vi "testExecution_Module.vi"(9 "Motion Cfg File path":path=path "C:/Users/Public/Documents/UCAR/APAR Board Test/SupportFiles/Motion64.ini", 10 "Cfg File path":path=path "C:/Users/Public/Documents/UCAR/APAR Board Test/SupportFiles/aparConfig.ini", 11 "MessageQues":T1) -> ()   [LabVIEW 2019]
doc: "This VI is a simple state machine that has a message que so it can be controlled by external processes.\nIt also has a control with all the messages ques in the calling application that it needs to send messages to.\n\nThe concept is to have many parallel VIs like this one. This VI should be a cohesive process. This could cut down on it's size and complexity.\n\nBolder Software LLC"
uses:
  Support/MessageQue/VXM Main Test App/MultipleMessageQues vxm.ctl
  Support/MessageQue/MessageQue.ctl
  Support/MessageQue/MessageCluster.ctl
  Classes/aparCfg/aparCfg.lvclass
  Classes/ArrayController/ArrayController.lvclass
  Classes/CopperMountain/C4209 PNA.lvclass
  Classes/Sequence/Sequence.lvclass
  Classes/Datalog/DataLog.lvclass
  Classes/SendMessage/SendMessage.lvclass
  Classes/MotionComm/MotionComm.lvclass
  UI temporary dialogs and VIs/Mode1TestProperties.ctl
  Classes/Sequence/SequenceSubvis/RF Direction.ctl
  Classes/DataLogRaster/DataLogRaster.lvclass
  C:/Users/MWUser/Desktop/GItHub/mmWave_Scanner/LVSource/Classes/Datalog/DataLog.lvclass
  VXM Public API/mmWaveAxis.ctl
  UI temporary dialogs and VIs/Mode2TestProperties.ctl
  UI temporary dialogs and VIs/Mode3TestProperties.ctl
  Support/MessageAPI/UIMessage.ctl
  Support/MessageQue/MessageQue.lvlib
  Classes/FileMerge/FileMerge.lvclass
  Classes/VXMCfg/VXMCfg.lvclass
panel:
  out "Seq Step":string
  out "i":i32
  out "Command":string
  out "error out":errorcluster
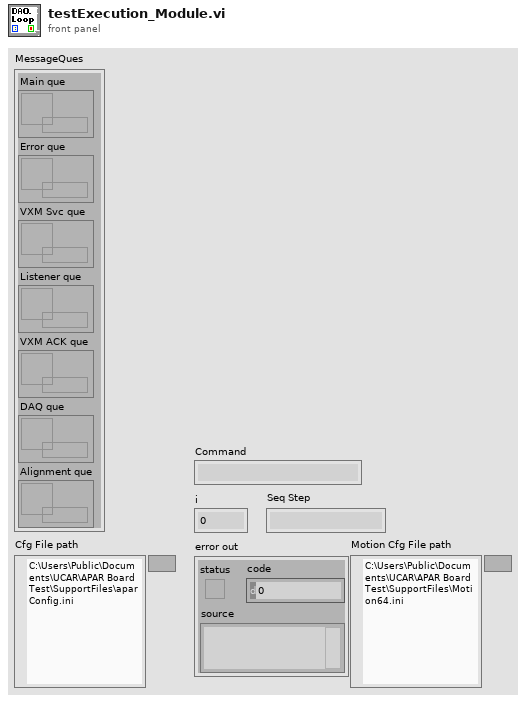
[diagram p1: front panel]
types:
  T1 = typedef "MultipleMessageQues vxm.ctl" = cluster{"Main que":T2, "Error que":T2, "VXM Svc que":T2, "Listener que":T2, "VXM ACK que":T2, "DAQ que":T2, "Alignment que":T2}
  T2 = typedef "MessageQue.lvlib/MessageQue.ctl" = refnum<queue>
  T3 = cluster{"aparCfg":refnum<class "aparCfg.lvclass">, "AC":refnum<class "ArrayController.lvclass">, "PNA":refnum<class "C4209 PNA.lvclass">, "Sequence":refnum<class "Sequence.lvclass">, "DataLog":refnum<class "DataLog.lvclass">, "UI Msg":refnum<class "SendMessage.lvclass">, "Motion ACK":refnum<class "MotionComm.lvclass">}
  T4 = typedef "UIMessage.ctl" = cluster{"EventCode":i32, "Numeric":dbl, "String":string, "Variant":variant}
  T5 = typedef "ACConfig.ctl" = cluster{"Board 1 alias":string, "Board 1 Enable":bool, "Board 2 alias":string, "Board 2 Enable":bool}
  T6 = typedef "N5222AConfig.ctl" = cluster{"ResourceName":string, "Enable":bool, "Channel":i32, "CalFileName":string, "MeasName":string, "TempDatFile":string, "Power, dBm":dbl, "NumPoints":i32, "Start Freq, Hz":dbl, "Stop Freq, Hz":dbl, "NumAverages":i32, "Sweep Type":i32, "IF Bandwidth":dbl}
  T7 = typedef "seqConfig.ctl" = cluster{"TempXMLFilePath":path, "Motion":bool}
  T8 = typedef "RunTest.ctl" = cluster{"FileNameRoot":string, "MergeFilePath":path, "Merge":bool}
  T9 = typedef "DataLogConfig.ctl" = cluster{"FilePath":path}
  T10 = typedef "sub-syst.n.ctl" = cluster{"Addr":string, "Enable":bool, "X scale eng./step":dbl, "Y scale eng./step":dbl, "Z scale eng./step":dbl, "T scale eng./step":dbl, "X units":string, "Y units":string, "Z units":string, "T units":string, "X Jog":dbl, "Y Jog":dbl, "Z Jog":dbl, "T Jog":dbl, "X-1 Name":string, "Y-2 Name":string, "Z-3 Name":string, "T-4 Name":string, "VXM (1-4)":i32}
  T11 = typedef "mmWaveAxis.ctl" = string
  T12 = typedef "Mode1TestProperties.ctl" = cluster{"Probe Horizontal Polarization":bool, "Probe Vertical Polarization":bool, "Data File Name":string, "RF In/Out of antenna":T13, "Raster XY Points":cluster{"X mm":dbl, "Y mm":dbl}[]}
  T13 = typedef "RF Direction.ctl" = enum16{"Tx - RF In", "Rx - RF Out"}
  T14 = typedef "Mode2TestProperties.ctl" = cluster{"Probe Horizontal Polarization":bool, "Probe Vertical Polarization":bool, "Upload TR Module file":path, "Data File Name":string, "RF In/Out of antenna":T13, "RT3 Positions, degrees":dbl[]}
  T15 = typedef "Mode3TestProperties.ctl" = cluster{"Probe Horizontal Polarization":bool, "Probe Vertical Polarization":bool, "Upload TR Module file":path, "Data File Name":string, "RF In/Out of antenna":T13}
  T16 = typedef "DataLog.lvclass/SearchableTag.ctl" = cluster{"Module, 0-63":i32, "RF Direction Tx0":T13, "Polarization, V0 H1":T17, "AO-64 Array":dbl[]}
  T17 = typedef "PolarizationSelect.ctl" = enum16{"Vertical", "Horizontal"}
  T18 = typedef "PatchNewTestStep.ctl" = cluster{"RF In/Out":T13, "TR Module/Raster":i32, "Polarization":T17, "Position":T19[]}
  T19 = typedef "singleAxisMoveDef.ctl" = cluster{"mmWave Axis":T11, "eng. value":dbl}
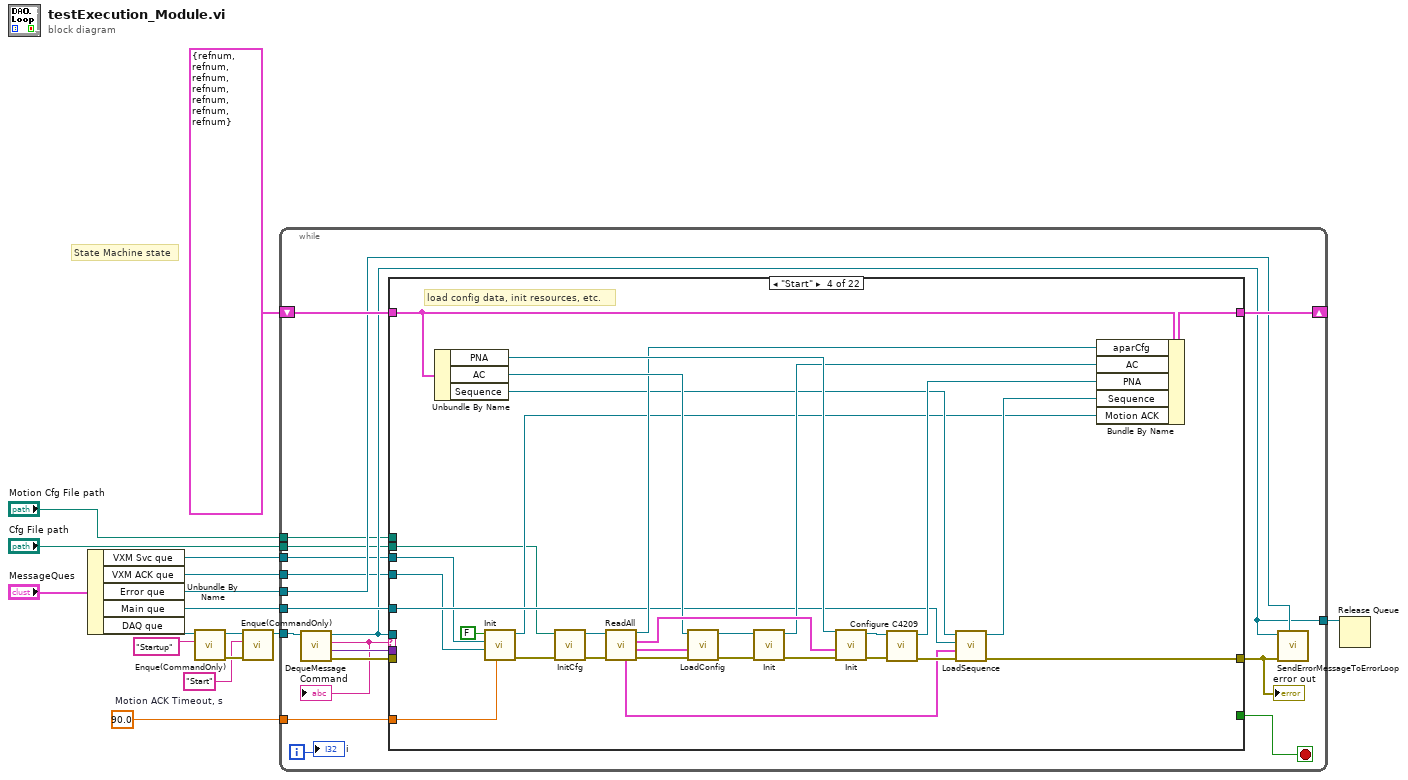
[diagram p0: block diagram]
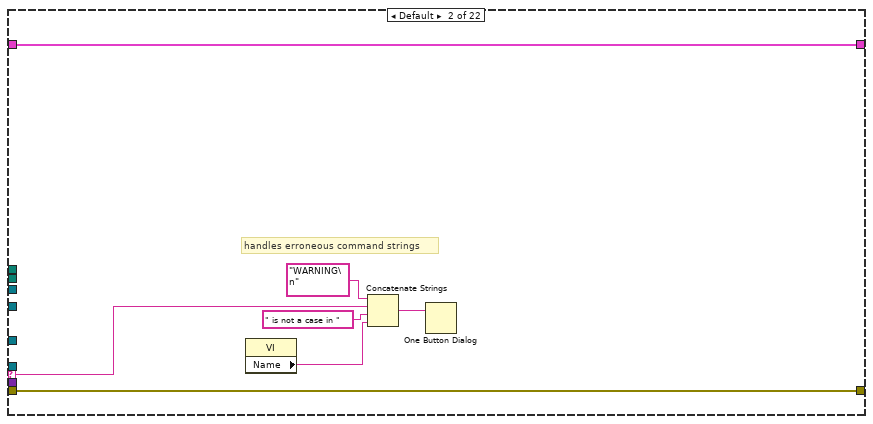
[diagram p3: hidden frame]
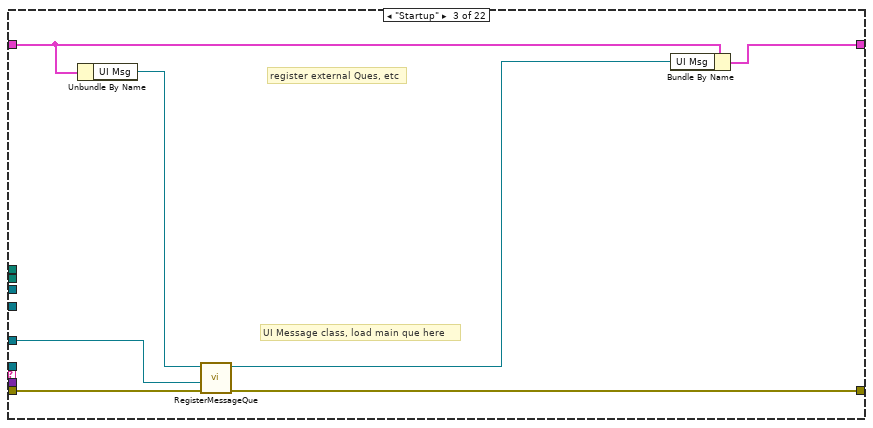
[diagram p4: hidden frame]
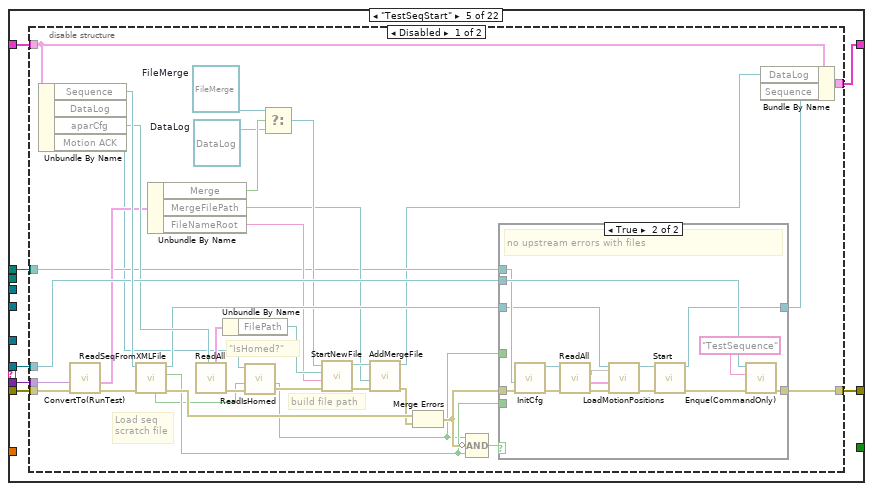
[diagram p5: hidden frame]
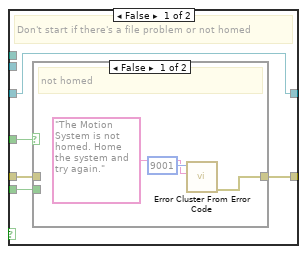
[diagram p6: hidden frame]
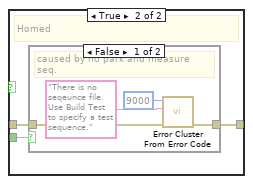
[diagram p7: hidden frame]
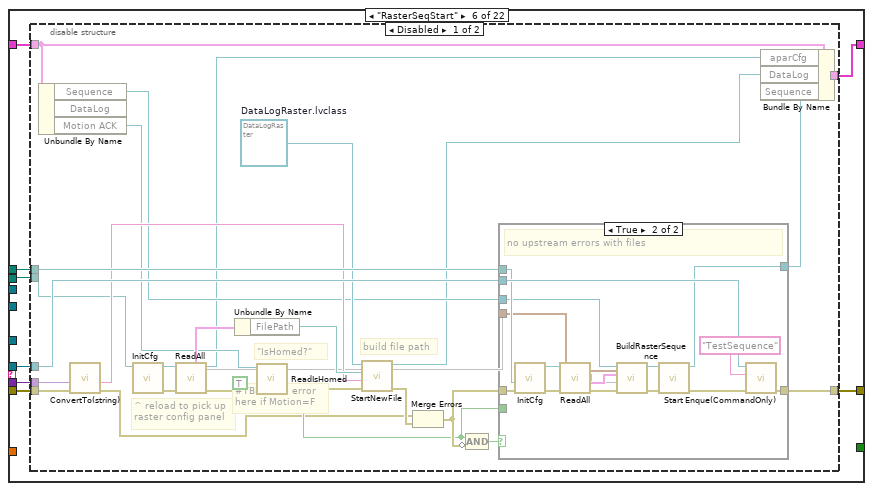
[diagram p10: hidden frame]
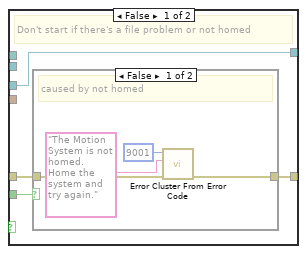
[diagram p11: hidden frame]
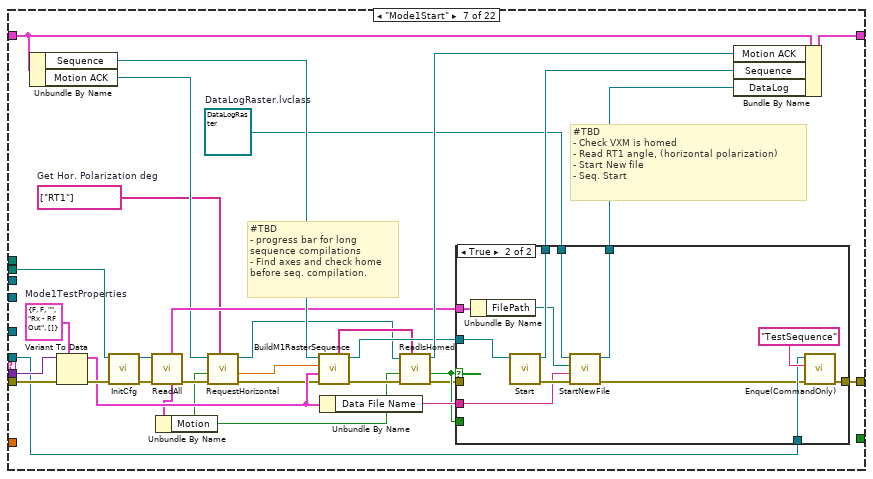
[diagram p14: hidden frame]
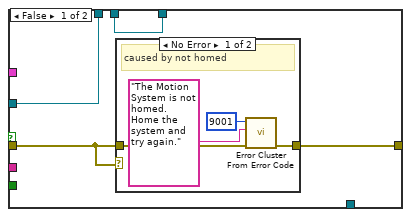
[diagram p15: hidden frame]
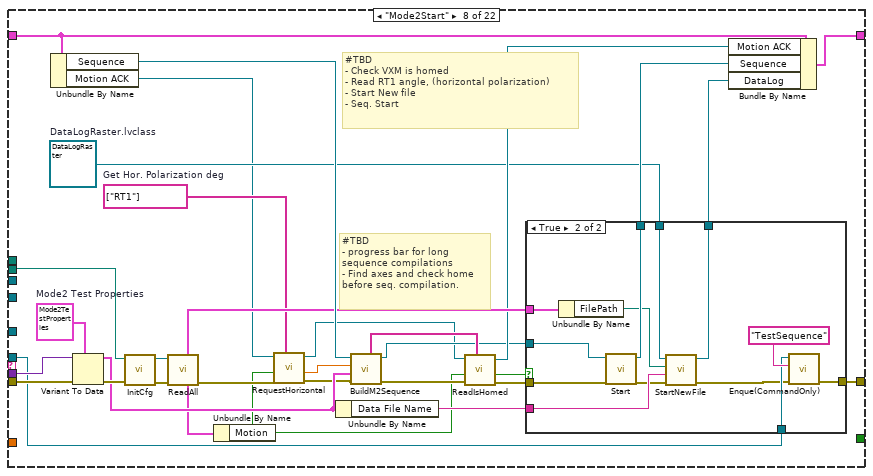
[diagram p17: hidden frame]
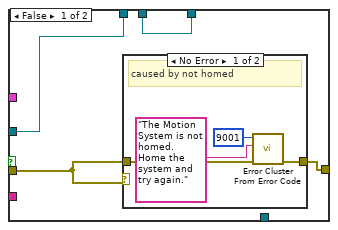
[diagram p18: hidden frame]
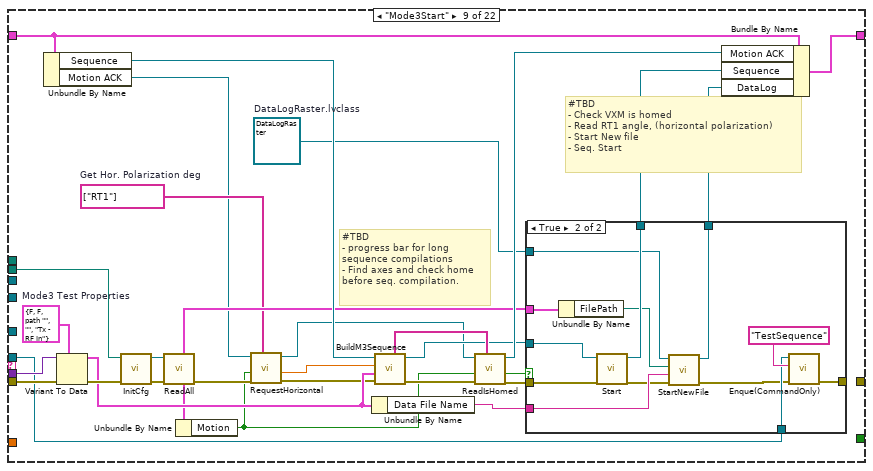
[diagram p20: hidden frame]
diagram:
  w2 = 90.0  # Motion ACK Timeout, s
  # "State Machine state"
  n1 = Unbundle By Name("MessageQues") -> ("VXM Svc que"=w4:T2, "VXM ACK que"=w3:T2, "Error que"=w14:T2, "Main que"=w15:T2, "DAQ que"=w12:T2)
  n2 = call "Enque(CommandOnly).vi"("Message Command"="Startup" ("Command"), "Message que"=w12) -> ("error out"=w9:errorcluster, "Message que out"=w8:T2)  [unwired: 8 in]
  n3 = call "Enque(CommandOnly).vi"("error in"=w9, "Message Command"="Start", "Message que"=w8) -> ("Message que out"=w7:T2)  [unwired: 7 in, 1 out]
  n4 = while {
    tunnel: w7 -> [w33]
    tunnel: w15 -> [w32]
    tunnel: w14 -> [w23]
    tunnel: [w22] -> w13
    shift-right: [w28] -> _
    shift-left: T3 {"aparCfg"=refnum, "AC"=refnum, "PNA"=refnum, "Sequence"=refnum, "DataLog"=refnum, "UI Msg"=refnum, "Motion ACK"=refnum} -> [w27]
    tunnel: "Cfg File path" -> [w21]
    tunnel: w4 -> [w20]
    tunnel: w3 -> [w19]
    tunnel: w2 -> [w18]
    tunnel: "Motion Cfg File path" -> [w17]
    i -> [w26]
    stop <- w30 stop-if-true
    n5 = call "DequeMessage.vi"("Message que"=w33) -> ("error out"=w31:errorcluster, "Message Payload"=w29:variant, "Message Command"=w25:string, "Message que out"=w22:T2)  [unwired: 5 in, 2 out]
    "Command" <- w25
    n6 = case shown="\"Start\"" w25 {
      selector: w25 -> [_ w36 _ _ _ _ _ _ _ _ _ _ _ _ _ _ _ _ _ _ _ _]
      tunnel: w32 -> [_ _ w43 w56 _ _ _ _ _ _ _ _ _ _ _ _ _ _ _ _ _ _]
      tunnel: w22 -> [_ _ _ _ w84 w158 w238 w292 w336 w395 w499 w512 w526 w536 _ _ _ _ _ _ _ _]
      tunnel: [_ w41 w47 w60 w85 w159 w237 w291 _ w396 w505 w514 w533 w538 _ w548 w561 w566 w578 _ w588 _] -> w24
      tunnel: w31 -> [_ w41 w42 _ w80 w154 w245 w298 w351 w381 w500 w515 w532 w537 _ w547 w563 w570 w578 _ _ _]
      tunnel: [_ _ _ _ _ _ _ _ _ _ _ _ _ _ _ _ _ _ _ _ _ TRUE] -> w30
      tunnel: w29 -> [_ _ _ _ w81 w155 w244 w297 w350 _ _ _ _ _ _ _ w562 w574 _ _ w587 _]
      tunnel: [w34 w40 w45 w69 w82 w156 w240 w294 w346 w391 w504 w519 w535 w545 w546 w550 w564 w568 w576 w585 w589 w590] -> w28
      tunnel: w27 -> [w34 w40 w46 w70 w83 w157 w242 w295 w348 w392 w502 w517 w534 w545 w546 w551 w565 w569 w577 w586 w589 w590]
      tunnel: w21 -> [_ _ _ w49 _ w152 w234 w284 w341 _ _ _ _ _ _ _ _ _ _ _ _ _]
      tunnel: w20 -> [_ _ _ w52 _ _ _ _ _ _ _ _ _ _ _ _ _ _ _ _ _ _]
      tunnel: w19 -> [_ _ _ w51 _ _ _ _ _ _ _ _ _ _ _ _ _ _ _ _ _ _]
      tunnel: w18 -> [_ _ _ w50 _ _ _ _ _ _ _ _ _ _ _ _ _ _ _ _ _ _]
      tunnel: w17 -> [_ _ _ _ w79 w153 _ _ _ _ _ _ _ _ _ _ _ _ _ _ _ _]
      frame "idle" {
      }
      frame Default {
        # "handles erroneous command strings"
        n7 = property class="VI"() -> ("Name"=w35:string)  [unwired: 2 in, 2 out]
        n8 = Concatenate Strings("WARNING\n" ("message"), w36, " is not a case in " ("message"), w35) -> (w39:string)
        n9 = One Button Dialog(message=w39) -> ()  [unwired: 1 in, 1 out]
      }
      frame "Startup" {
        # "UI Message class, load main que here"
        # "register external Ques, etc"
        n10 = Unbundle By Name(w46) -> ("UI Msg"=w48:refnum<class "SendMessage.lvclass">)
        n11 = call "RegisterMessageQue.vi"("error in (no error)"=w42, "Message que"=w43, "SendMessage in"=w48) -> ("error out"=w47:errorcluster, "SendMessage out"=w44:refnum<class "SendMessage.lvclass">)  [unwired: 7 in]
        n12 = Bundle By Name(cluster=w46, "UI Msg"=w44) -> (w45:T3)
      }
      frame "Start" {
        # "load config data, init resources, etc."
        n13 = Unbundle By Name(w70) -> ("PNA"=w71:refnum<class "C4209 PNA.lvclass">, "AC"=w72:refnum<class "ArrayController.lvclass">, "Sequence"=w59:refnum<class "Sequence.lvclass">)
        n14 = call "Init.vi"("Timeout, s"=w50, "VXM ACK que"=w51, "VXM Svc que"=w52, "Standalone"=FALSE) -> ("error out"=w55:errorcluster, "MotionComm out"=w54:refnum<class "MotionComm.lvclass">)  [unwired: 6 in]
        n15 = call "InitCfg.vi"("error in (no error)"=w55, "Cfg File path"=w49) -> ("error out"=w65:errorcluster, "aparCfg out"=w66:refnum<class "aparCfg.lvclass">)  [unwired: 8 in]
        n16 = call "ReadAll.vi"("error in (no error)"=w65, "aparCfg in"=w66) -> ("error out"=w74:errorcluster, "ACConfig"=w78:T5, "N5222A Cfg"=w76:T6, "aparCfg out"=w68:refnum<class "aparCfg.lvclass">, "SequenceConfig"=w57:T7)  [unwired: 4 in, 1 out]
        n17 = call "LoadConfig.vi"("error in (no error)"=w74, "AC Config"=w78, "ArrayController in"=w72) -> ("error out"=w77:errorcluster, "ArrayController out"=w73:refnum<class "ArrayController.lvclass">)  [unwired: 7 in]
        n18 = call "Init.vi"("error in (no error)"=w77, "ArrayController in"=w73) -> ("error out"=w75:errorcluster, "ArrayController out"=w67:refnum<class "ArrayController.lvclass">)  [unwired: 8 in]
        n19 = call "Init.vi"("error in (no error)"=w75, "C4209 Cfg"=w76, "C4209 PNA"=w71) -> ("error out"=w62:errorcluster, "C4209 PNA out"=w64:refnum<class "C4209 PNA.lvclass">)  [unwired: 7 in]
        n20 = call "Configure C4209.vi"("error in (no error)"=w62, "C4209 PNA"=w64) -> ("error out"=w61:errorcluster, "C4209 PNA out"=w63:refnum<class "C4209 PNA.lvclass">)  [unwired: 8 in]
        n21 = call "LoadSequence.vi"("error in (no error)"=w61, "Sequence Cfg"=w57, "Message que"=w56, "Sequence in"=w59) -> ("error out"=w60:errorcluster, "Sequence out"=w58:refnum<class "Sequence.lvclass">)  [unwired: 6 in]
        n22 = Bundle By Name(cluster=w70, "aparCfg"=w68, "AC"=w67, "PNA"=w63, "Sequence"=w58, "Motion ACK"=w54) -> (w69:T3)
      }
      frame "TestSeqStart" {
        n23 = disable-structure shown="Disabled" {
          disable-tunnel: [w119 _] -> w85
          disable-tunnel: w84 -> [w117 _]
          disable-tunnel: w83 -> [w116 w151]
          disable-tunnel: [w115 w151] -> w82
          disable-tunnel: w81 -> [w114 _]
          disable-tunnel: w80 -> [w113 _]
          disable-tunnel: w79 -> [w92 _]
          frame Disabled {
            w100 = refnum<class "FileMerge.lvclass"> refnum  # FileMerge
            w99 = refnum<class "DataLog.lvclass"> refnum  # DataLog
            # "\"IsHomed?\""
            # "build file path"
            # "Load seq \nscratch file"
            n24 = Unbundle By Name(w116) -> ("Sequence"=w118:refnum<class "Sequence.lvclass">, "aparCfg"=w111:refnum<class "aparCfg.lvclass">, "Motion ACK"=w88:refnum<class "MotionComm.lvclass">)  [unwired: 1 out]
            n25 = call "ConvertTo(RunTest).vi"("error in"=w113, "Message Payload"=w114) -> ("error out"=w112:errorcluster, "RunTest"=w110:T8)  [unwired: 8 in]
            n26 = call "ReadSeqFromXMLFile.vi"("error in (no error)"=w112, "Sequence in"=w118) -> ("error out"=w107:errorcluster, "Valid Seq"=w103:bool, "Sequence out"=w106:refnum<class "Sequence.lvclass">, "Motion"=w86:bool)  [unwired: 5 in, 1 out]
            n27 = Unbundle By Name(w110) -> ("Merge"=w101:bool, "MergeFilePath"=w93:path, "FileNameRoot"=w94:string)
            n28 = call "ReadAll.vi"("aparCfg in"=w111) -> ("error out"=w90:errorcluster, "DataLogConfig"=w109:T9)  [unwired: 5 in, 4 out]
            n29 = Unbundle By Name(w109) -> ("FilePath"=w108:path)
            n30 = call "ReadIsHomed.vi"("error in (no error)"=w90, "Motion Config"=w86, "MotionComm in"=w88) -> ("error out"=w89:errorcluster, "True = Homed"=w87:bool)  [unwired: 6 in, 1 out]
            n31 = Select(t=w100, s=w101, f=w99) -> (s? t:f=w98:refnum<class "DataLog.lvclass">)
            n32 = call-dynamic "StartNewFile.vi"("error in (no error)"=w89, "Root File Name"=w94, "Data Files Folder Path"=w108, "DataLog in"=w98) -> ("error out"=w97:errorcluster, "DataLog out"=w95:refnum<class "DataLog.lvclass">)  [unwired: 6 in]
            n33 = call-dynamic "AddMergeFile.vi"("error in (no error)"=w97, "ExistingFilePath"=w93, "DataLog in"=w95) -> ("error out"=w96:errorcluster, "DataLog out"=w91:refnum<class "DataLog.lvclass">)  [unwired: 7 in]
            n34 = Merge Errors(w107, w96) -> (w105:errorcluster)
            n35 = Compound Arithmetic op=AND(w87, invert w105, w103) -> (w104:bool)
            n36 = case shown="True" w104 {
              tunnel: [w123 w150] -> w119
              tunnel: w117 -> [_ w149]
              tunnel: w105 -> [w124 w144]
              tunnel: w106 -> [w121 w138]
              tunnel: [w121 w146] -> w102
              tunnel: w103 -> [w122 _]
              tunnel: w92 -> [_ w142]
              tunnel: w87 -> [w120 _]
              frame False {
                # "Don't start if there's a file problem or not homed"
                n37 = case shown="False" w120 {
                  tunnel: w124 -> [_ w130]
                  tunnel: [w125 w129] -> w123
                  tunnel: w122 -> [_ w128]
                  frame False {
                    # "not homed"
                    n38 = call <vilib>:"Error Cluster From Error Code.vi"("error message (\"\")"="The Motion System is not homed. Home the system and try again." ("error message (\"\")"), "error code (0)"=9001) -> ("error out"=w125:errorcluster)  [unwired: 7 in]
                  }
                  frame True {
                    # "Homed"
                    n39 = case shown="False" w128 {
                      tunnel: w130 -> [w134 w135]
                      tunnel: [w133 w135] -> w129
                      frame False {
                        # "caused by no park and measure seq."
                        n40 = call <vilib>:"Error Cluster From Error Code.vi"("error in (no error)"=w134, "error message (\"\")"="There is no seqeunce file. Use Build Test to specify a test sequence." ("error message (\"\")"), "error code (0)"=9000) -> ("error out"=w133:errorcluster)  [unwired: 6 in]
                      }
                      frame True {
                        # "pass through error"
                      }
                    }
                  }
                }
              }
              frame True {
                # "no upstream errors with files"
                n41 = call "InitCfg.vi"("error in (no error)"=w144, "Cfg File path"=w142) -> ("error out"=w143:errorcluster, "VXMCfg out"=w145:refnum<class "VXMCfg.lvclass">)  [unwired: 7 in, 1 out]
                n42 = call "ReadAll.vi"("error in (no error)"=w143, "VXMCfg in"=w145) -> ("error out"=w141:errorcluster, "VXM Properties.sub-syst.3"=w137:T10, 10:w136)  [unwired: 4 in, 3 out]
                n43 = call "LoadMotionPositions.vi"("TestZT"=w136, "error in (no error)"=w141, "Position Array"=w137, "Sequence in"=w138) -> ("error out"=w140:errorcluster, "Sequence out"=w139:refnum<class "Sequence.lvclass">)  [unwired: 6 in]
                n44 = call "Start.vi"("error in (no error)"=w140, "Sequence in"=w139) -> ("error out"=w147:errorcluster, "Sequence out"=w146:refnum<class "Sequence.lvclass">)  [unwired: 8 in]
                n45 = call "Enque(CommandOnly).vi"("error in"=w147, "Message Command"="TestSequence" ("Command"), "Message que"=w149) -> ("error out"=w150:errorcluster)  [unwired: 7 in, 1 out]
              }
            }
            n46 = Bundle By Name(cluster=w116, "DataLog"=w91, "Sequence"=w102) -> (w115:T3)
          }
          frame Enabled {
          }
        }
      }
      frame "RasterSeqStart" {
        n47 = disable-structure shown="Disabled" {
          disable-tunnel: [w187 _] -> w159
          disable-tunnel: w158 -> [w186 _]
          disable-tunnel: w157 -> [w185 w213]
          disable-tunnel: [w184 w213] -> w156
          disable-tunnel: w155 -> [w183 _]
          disable-tunnel: w154 -> [w182 _]
          disable-tunnel: w153 -> [w176 _]
          disable-tunnel: w152 -> [w164 _]
          frame Disabled {
            w172 = refnum<class "DataLogRaster.lvclass"> refnum  # DataLogRaster.lvclass
            # "#TBD need error here if Motion=F"
            # "^ reload to pick up\nraster config panel"
            # "\"IsHomed?\""
            # "build file path"
            n48 = Unbundle By Name(w185) -> ("Sequence"=w169:refnum<class "Sequence.lvclass">, "Motion ACK"=w165:refnum<class "MotionComm.lvclass">)  [unwired: 1 out]
            n49 = call "ConvertTo(string).vi"("error in"=w182, "Message Payload"=w183) -> ("error out"=w161:errorcluster, "Message Payload string"=w173:string)  [unwired: 8 in]
            n50 = call "InitCfg.vi"("Cfg File path"=w164) -> ("error out"=w162:errorcluster, "aparCfg out"=w166:refnum<class "aparCfg.lvclass">)  [unwired: 9 in]
            n51 = call "ReadAll.vi"("error in (no error)"=w162, "aparCfg in"=w166) -> ("error out"=w175:errorcluster, "aparCfg out"=w163:refnum<class "aparCfg.lvclass">, "DataLogConfig"=w181:T9, 7:w168)  [unwired: 3 in, 3 out]
            n52 = Unbundle By Name(w181) -> ("FilePath"=w180:path)
            n53 = call "ReadIsHomed.vi"("error in (no error)"=w175, "Motion Config"=TRUE, "MotionComm in"=w165) -> ("error out"=w174:errorcluster, "True = Homed"=w170:bool)  [unwired: 6 in, 1 out]
            n54 = call-dynamic "StartNewFile.vi"("error in (no error)"=w174, "Root File Name"=w173, "Data Files Folder Path"=w180, "DataLogRaster in"=w172) -> ("error out"=w171:errorcluster, "DataLogRaster out"=w167:refnum<class "DataLogRaster.lvclass">)  [unwired: 6 in]
            n55 = Merge Errors(w161, w171) -> (w179:errorcluster)
            n56 = Compound Arithmetic op=AND(w170, invert w179) -> (w178:bool)
            n57 = case shown="True" w178 {
              tunnel: [w190 w212] -> w187
              tunnel: w186 -> [_ w211]
              tunnel: w179 -> [w191 w208]
              tunnel: w169 -> [w188 w204]
              tunnel: [w188 w197] -> w177
              tunnel: w170 -> [w189 _]
              tunnel: w176 -> [_ w206]
              tunnel: w168 -> [_ w201]
              frame False {
                # "Don't start if there's a file problem or not homed"
                n58 = case shown="False" w189 {
                  tunnel: w191 -> [w195 w196]
                  tunnel: [w194 w196] -> w190
                  frame False {
                    # "caused by not homed"
                    n59 = call <vilib>:"Error Cluster From Error Code.vi"("error in (no error)"=w195, "error message (\"\")"="The Motion System is not homed. Home the system and try again." ("error message (\"\")"), "error code (0)"=9001) -> ("error out"=w194:errorcluster)  [unwired: 6 in]
                  }
                  frame True {
                    # "pass through error"
                  }
                }
              }
              frame True {
                # "no upstream errors with files"
                n60 = call "InitCfg.vi"("error in (no error)"=w208, "Cfg File path"=w206) -> ("error out"=w207:errorcluster, "VXMCfg out"=w209:refnum<class "VXMCfg.lvclass">)  [unwired: 7 in, 1 out]
                n61 = call "ReadAll.vi"("error in (no error)"=w207, "VXMCfg in"=w209) -> ("error out"=w205:errorcluster, "VXM Properties.sub-syst.3"=w203:T10, 10:w202)  [unwired: 4 in, 3 out]
                n62 = call "BuildRasterSequence.vi"("RasterDef"=w201, "error in (no error)"=w205, "TestZT"=w202, "Position Array in"=w203, "Sequence in"=w204) -> ("error out"=w199:errorcluster, "Sequence out"=w200:refnum<class "Sequence.lvclass">)  [unwired: 4 in, 1 out]
                n63 = call "Start.vi"("error in (no error)"=w199, "Sequence in"=w200) -> ("error out"=w198:errorcluster, "Sequence out"=w197:refnum<class "Sequence.lvclass">)  [unwired: 8 in]
                n64 = call "Enque(CommandOnly).vi"("error in"=w198, "Message Command"="TestSequence" ("Command"), "Message que"=w211) -> ("error out"=w212:errorcluster)  [unwired: 7 in, 1 out]
              }
            }
            n65 = Bundle By Name(cluster=w185, "aparCfg"=w163, "DataLog"=w167, "Sequence"=w177) -> (w184:T3)
          }
          frame Enabled {
          }
        }
      }
      frame "Mode1Start" {
        w214 = T11[] ["RT1"]  # Get Hor. Polarization deg
        w221 = refnum<class "DataLogRaster.lvclass"> refnum  # DataLogRaster.lvclass
        w243 = T12 {"Probe Horizontal Polarization"=FALSE, "Probe Vertical Polarization"=FALSE, "Data File Name"="", "RF In/Out of antenna"=enum."Rx - RF Out", "Raster XY Points"=[]}  # Mode1TestProperties
        # "#TBD\n- progress bar for long\nsequence compilations\n- Find axes and check home\nbefore seq. compilation."
        # "#TBD\n- Check VXM is homed\n- Read RT1 angle, (horizontal polarization)\n- Start New file\n- Seq. Start"
        n66 = Unbundle By Name(w242) -> ("Sequence"=w241:refnum<class "Sequence.lvclass">, "Motion ACK"=w217:refnum<class "MotionComm.lvclass">)
        n67 = Variant To Data(error in=w245, type=w243, Variant=w244) -> (data=w232:T12, error out=w233:errorcluster)
        n68 = call "InitCfg.vi"("error in (no error)"=w233, "Cfg File path"=w234) -> ("error out"=w235:errorcluster, "aparCfg out"=w236:refnum<class "aparCfg.lvclass">)  [unwired: 8 in]
        n69 = call "ReadAll.vi"("error in (no error)"=w235, "aparCfg in"=w236) -> ("error out"=w220:errorcluster, "SequenceConfig"=w229:T7, "DataLogConfig"=w224:T9)  [unwired: 4 in, 3 out]
        n70 = Unbundle By Name(w229) -> ("Motion"=w215:bool)
        n71 = call "RequestHorizontal.vi"("check postion of these axes"=w214, "error in (no error)"=w220, "Motion Config"=w215, "MotionComm in"=w217) -> ("error out"=w219:errorcluster, "Horizontal polarization position"=w218:dbl, "MotionComm out"=w216:refnum<class "MotionComm.lvclass">)  [unwired: 5 in]
        n72 = call "BuildM1RasterSequence.vi"("error in (no error)"=w219, "Mode3TestProperties"=w232, "Horizontal T deg"=w218, "Sequence in"=w241) -> ("error out"=w226:errorcluster, "Sequence out"=w227:refnum<class "Sequence.lvclass">, "Axes to Move"=w225:T11[])  [unwired: 4 in, 1 out]
        n73 = Unbundle By Name(w232) -> ("Data File Name"=w231:string)
        n74 = call "ReadIsHomed.vi"("check these axes homed"=w225, "error in (no error)"=w226, "Motion Config"=w215, "MotionComm in"=w216) -> ("error out"=w222:errorcluster, "True = Homed"=w223:bool, "MotionComm out"=w228:refnum<class "MotionComm.lvclass">)  [unwired: 5 in]
        n75 = case shown="True" w223 {
          tunnel: [w248 w265] -> w239
          tunnel: w238 -> [_ w264]
          tunnel: [w247 w263] -> w237
          tunnel: w221 -> [w249 w262]
          tunnel: w231 -> [_ w259]
          tunnel: [w249 w258] -> w230
          tunnel: w223 -> [_ _]
          tunnel: w227 -> [w248 w257]
          tunnel: w224 -> [_ w256]
          tunnel: w222 -> [w246 _]
          frame False {
            n76 = case shown="No Error" w246 {
              tunnel: w246 -> [w253 w254]
              tunnel: [w252 w254] -> w247
              frame No Error {
                # "caused by not homed"
                n77 = call <vilib>:"Error Cluster From Error Code.vi"("error in (no error)"=w253, "error message (\"\")"="The Motion System is not homed. Home the system and try again." ("error message (\"\")"), "error code (0)"=9001) -> ("error out"=w252:errorcluster)  [unwired: 6 in]
              }
              frame Error {
                # "pass through error"
              }
            }
          }
          frame True {
            n78 = Unbundle By Name(w256) -> ("FilePath"=w260:path)
            n79 = call "Start.vi"("Sequence in"=w257) -> ("error out"=w261:errorcluster, "Sequence out"=w265:refnum<class "Sequence.lvclass">)  [unwired: 9 in]
            n80 = call-dynamic "StartNewFile.vi"("error in (no error)"=w261, "Root File Name"=w259, "Data Files Folder Path"=w260, "DataLogRaster in"=w262) -> ("error out"=w255:errorcluster, "DataLogRaster out"=w258:refnum<class "DataLogRaster.lvclass">)  [unwired: 6 in]
            n81 = call "Enque(CommandOnly).vi"("error in"=w255, "Message Command"="TestSequence" ("Command"), "Message que"=w264) -> ("error out"=w263:errorcluster)  [unwired: 7 in, 1 out]
          }
        }
        n82 = Bundle By Name(cluster=w242, "Motion ACK"=w228, "Sequence"=w239, "DataLog"=w230) -> (w240:T3)
      }
      frame "Mode2Start" {
        w273 = T11[] ["RT1"]  # Get Hor. Polarization deg
        w275 = refnum<class "DataLogRaster.lvclass"> refnum  # DataLogRaster.lvclass
        w296 = T14 {"Probe Horizontal Polarization"=FALSE, "Probe Vertical Polarization"=FALSE, "Upload TR Module file"=path "", "Data File Name"="", "RF In/Out of antenna"=enum."Tx - RF In", "RT3 Positions, degrees"=[]}  # Mode2 Test Properties
        # "#TBD\n- progress bar for long\nsequence compilations\n- Find axes and check home\nbefore seq. compilation."
        # "#TBD\n- Check VXM is homed\n- Read RT1 angle, (horizontal polarization)\n- Start New file\n- Seq. Start"
        n83 = Unbundle By Name(w295) -> ("Sequence"=w293:refnum<class "Sequence.lvclass">, "Motion ACK"=w270:refnum<class "MotionComm.lvclass">)
        n84 = Variant To Data(error in=w298, type=w296, Variant=w297) -> (data=w283:T14, error out=w285:errorcluster)
        n85 = call "InitCfg.vi"("error in (no error)"=w285, "Cfg File path"=w284) -> ("error out"=w288:errorcluster, "aparCfg out"=w289:refnum<class "aparCfg.lvclass">)  [unwired: 8 in]
        n86 = call "ReadAll.vi"("error in (no error)"=w288, "aparCfg in"=w289) -> ("error out"=w272:errorcluster, "SequenceConfig"=w281:T7, "DataLogConfig"=w287:T9)  [unwired: 4 in, 3 out]
        n87 = Unbundle By Name(w281) -> ("Motion"=w268:bool)
        n88 = call "RequestHorizontal.vi"("check postion of these axes"=w273, "error in (no error)"=w272, "Motion Config"=w268, "MotionComm in"=w270) -> ("error out"=w271:errorcluster, "Horizontal polarization position"=w267:dbl, "MotionComm out"=w269:refnum<class "MotionComm.lvclass">)  [unwired: 5 in]
        n89 = Unbundle By Name(w283) -> ("Data File Name"=w286:string)
        n90 = call "BuildM2Sequence.vi"("error in (no error)"=w271, "Mode2 Test Properties"=w283, "Horizontal T deg"=w267, "Sequence in"=w293) -> ("error out"=w279:errorcluster, "Sequence out"=w276:refnum<class "Sequence.lvclass">, "Axes to Move"=w277:T11[])  [unwired: 4 in, 1 out]
        n91 = call "ReadIsHomed.vi"("check these axes homed"=w277, "error in (no error)"=w279, "Motion Config"=w268, "MotionComm in"=w269) -> ("error out"=w278:errorcluster, "True = Homed"=w274:bool, "MotionComm out"=w280:refnum<class "MotionComm.lvclass">)  [unwired: 5 in]
        n92 = case shown="True" w274 {
          tunnel: w292 -> [_ w319]
          tunnel: [w300 w318] -> w291
          tunnel: [w301 w317] -> w290
          tunnel: w287 -> [_ w316]
          tunnel: w286 -> [_ w314]
          tunnel: [w302 w312] -> w282
          tunnel: w278 -> [w299 w311]
          tunnel: w276 -> [w301 w310]
          tunnel: w275 -> [w302 w309]
          frame False {
            n93 = case shown="No Error" w299 {
              tunnel: w299 -> [w306 w307]
              tunnel: [w305 w307] -> w300
              frame No Error {
                # "caused by not homed"
                n94 = call <vilib>:"Error Cluster From Error Code.vi"("error in (no error)"=w306, "error message (\"\")"="The Motion System is not homed. Home the system and try again." ("error message (\"\")"), "error code (0)"=9001) -> ("error out"=w305:errorcluster)  [unwired: 6 in]
              }
              frame Error {
                # "pass through error"
              }
            }
          }
          frame True {
            n95 = Unbundle By Name(w316) -> ("FilePath"=w315:path)
            n96 = call "Start.vi"("error in (no error)"=w311, "Sequence in"=w310) -> ("error out"=w313:errorcluster, "Sequence out"=w317:refnum<class "Sequence.lvclass">)  [unwired: 8 in]
            n97 = call-dynamic "StartNewFile.vi"("error in (no error)"=w313, "Root File Name"=w314, "Data Files Folder Path"=w315, "DataLogRaster in"=w309) -> ("error out"=w308:errorcluster, "DataLogRaster out"=w312:refnum<class "DataLogRaster.lvclass">)  [unwired: 6 in]
            n98 = call "Enque(CommandOnly).vi"("error in"=w308, "Message Command"="TestSequence" ("Command"), "Message que"=w319) -> ("error out"=w318:errorcluster)  [unwired: 7 in, 1 out]
          }
        }
        n99 = Bundle By Name(cluster=w295, "Motion ACK"=w280, "Sequence"=w290, "DataLog"=w282) -> (w294:T3)
      }
      frame "Mode3Start" {
        w327 = T11[] ["RT1"]  # Get Hor. Polarization deg
        w332 = refnum<class "DataLogRaster.lvclass"> refnum  # DataLogRaster.lvclass
        w349 = T15 {"Probe Horizontal Polarization"=FALSE, "Probe Vertical Polarization"=FALSE, "Upload TR Module file"=path "", "Data File Name"="", "RF In/Out of antenna"=enum."Tx - RF In"}  # Mode3 Test Properties
        # "#TBD\n- progress bar for long\nsequence compilations\n- Find axes and check home\nbefore seq. compilation."
        # "#TBD\n- Check VXM is homed\n- Read RT1 angle, (horizontal polarization)\n- Start New file\n- Seq. Start"
        n100 = Unbundle By Name(w348) -> ("Sequence"=w347:refnum<class "Sequence.lvclass">, "Motion ACK"=w323:refnum<class "MotionComm.lvclass">)
        n101 = Variant To Data(error in=w351, type=w349, Variant=w350) -> (data=w342:T15, error out=w343:errorcluster)
        n102 = call "InitCfg.vi"("error in (no error)"=w343, "Cfg File path"=w341) -> ("error out"=w344:errorcluster, "aparCfg out"=w345:refnum<class "aparCfg.lvclass">)  [unwired: 8 in]
        n103 = call "ReadAll.vi"("error in (no error)"=w344, "aparCfg in"=w345) -> ("error out"=w326:errorcluster, "SequenceConfig"=w340:T7, "DataLogConfig"=w334:T9)  [unwired: 4 in, 3 out]
        n104 = Unbundle By Name(w340) -> ("Motion"=w322:bool)
        n105 = call "RequestHorizontal.vi"("check postion of these axes"=w327, "error in (no error)"=w326, "Motion Config"=w322, "MotionComm in"=w323) -> ("error out"=w325:errorcluster, "Horizontal polarization position"=w324:dbl, "MotionComm out"=w321:refnum<class "MotionComm.lvclass">)  [unwired: 5 in]
        n106 = Unbundle By Name(w342) -> ("Data File Name"=w335:string)
        n107 = call "BuildM3Sequence.vi"("error in (no error)"=w325, "Mode3 Test Properties"=w342, "Horizontal T deg"=w324, "Sequence in"=w347) -> ("error out"=w338:errorcluster, "Sequence out"=w333:refnum<class "Sequence.lvclass">, "Axes to Move"=w337:T11[])  [unwired: 4 in, 1 out]
        n108 = call "ReadIsHomed.vi"("check these axes homed"=w337, "error in (no error)"=w338, "Motion Config"=w322, "MotionComm in"=w321) -> ("error out"=w328:errorcluster, "True = Homed"=w331:bool, "MotionComm out"=w339:refnum<class "MotionComm.lvclass">)  [unwired: 5 in]
        n109 = case shown="True" w331 {
          tunnel: w336 -> [_ w372]
          tunnel: [w354 w371] -> _
          tunnel: [w355 w370] -> w330
          tunnel: w334 -> [_ w369]
          tunnel: w335 -> [_ w367]
          tunnel: [w352 w365] -> w329
          tunnel: w328 -> [w353 w364]
          tunnel: w333 -> [w355 w363]
          tunnel: w332 -> [w352 w361]
          frame False {
            n110 = case shown="No Error" w353 {
              tunnel: w353 -> [w359 w360]
              tunnel: [w358 w360] -> w354
              frame No Error {
                # "caused by not homed"
                n111 = call <vilib>:"Error Cluster From Error Code.vi"("error in (no error)"=w359, "error message (\"\")"="The Motion System is not homed. Home the system and try again." ("error message (\"\")"), "error code (0)"=9001) -> ("error out"=w358:errorcluster)  [unwired: 6 in]
              }
              frame Error {
                # "pass through error"
              }
            }
          }
          frame True {
            n112 = Unbundle By Name(w369) -> ("FilePath"=w368:path)
            n113 = call "Start.vi"("error in (no error)"=w364, "Sequence in"=w363) -> ("error out"=w366:errorcluster, "Sequence out"=w370:refnum<class "Sequence.lvclass">)  [unwired: 8 in]
            n114 = call-dynamic "StartNewFile.vi"("error in (no error)"=w366, "Root File Name"=w367, "Data Files Folder Path"=w368, "DataLogRaster in"=w361) -> ("error out"=w362:errorcluster, "DataLogRaster out"=w365:refnum<class "DataLogRaster.lvclass">)  [unwired: 6 in]
            n115 = call "Enque(CommandOnly).vi"("error in"=w362, "Message Command"="TestSequence" ("Command"), "Message que"=w372) -> ("error out"=w371:errorcluster)  [unwired: 7 in, 1 out]
          }
        }
        n116 = Bundle By Name(cluster=w348, "Motion ACK"=w339, "Sequence"=w330, "DataLog"=w329) -> (w346:T3)
      }
      frame "TestSequence" {
        n117 = Unbundle By Name(w392) -> ("Sequence"=w394:refnum<class "Sequence.lvclass">, "AC"=w387:refnum<class "ArrayController.lvclass">, "PNA"=w385:refnum<class "C4209 PNA.lvclass">, "DataLog"=w378:refnum<class "DataLog.lvclass">, "UI Msg"=w377:refnum<class "SendMessage.lvclass">, "Motion ACK"=w375:refnum<class "MotionComm.lvclass">)
        n118 = call "ExecuteSequence.vi"("Sequence in"=w394) -> ("Command"=w393:string, "SweepProperties"=w384:T16, "Sequence out"=w390:refnum<class "Sequence.lvclass">, "Sequence is done"=w382:bool, "Next Position"=w383:T18)  [unwired: 5 in, 1 out]
        "Seq Step" <- w393
        n119 = case shown="\"SweepTest\"" w393 {
          tunnel: [w422 w450 w467 w492] -> w389
          tunnel: w390 -> [w422 w450 w467 w492]
          tunnel: [w398 w427 w468 w491] -> w388
          tunnel: w387 -> [w400 w428 w468 w491]
          tunnel: [w419 w432 w463 w484] -> w386
          tunnel: w385 -> [w414 w444 w464 w485]
          tunnel: w384 -> [w404 w433 _ _]
          tunnel: w383 -> [w403 w434 w457 _]
          tunnel: w381 -> [w401 w429 _ w490]
          tunnel: [w412 w442 w466 w483] -> w380
          tunnel: [w415 w445 w465 w488] -> w379
          tunnel: w378 -> [w416 w446 w465 w489]
          tunnel: w377 -> [w411 w441 w462 w482]
          tunnel: [w410 w440 w462 w482] -> w376
          tunnel: w375 -> [w405 w435 w460 w481]
          tunnel: [w405 w435 w459 w481] -> w374
          frame "SweepTest" {
            n120 = call "d.vi"("error in (no error)"=w401, "d Cmd Properties"=w404, "ArrayController in"=w400) -> ("error out"=w418:errorcluster, "ArrayController out"=w398:refnum<class "ArrayController.lvclass">)  [unwired: 7 in]
            n121 = Unbundle By Name(w403) -> ("Position"=w402:T19[])
            n122 = flat-sequence {
              tunnel: [w423] -> w399
              tunnel: w418 -> [w423]
              frame #0 {
                n123 = Wait (ms)(milliseconds to wait=u32 10) -> ()  [unwired: 1 out]
              }
            }
            n124 = call "TriggerAndAveraging.vi"("error in (no error)"=w399, "C4209 PNA"=w414) -> ("error out"=w421:errorcluster, "C4209 PNA out"=w420:refnum<class "C4209 PNA.lvclass">)  [unwired: 8 in]
            n125 = call "SaveAndLoadTest.vi"("error in (no error)"=w421, "C4209 PNA"=w420) -> ("error out"=w417:errorcluster, "text"=w406:string, "C4209 PNA out"=w419:refnum<class "C4209 PNA.lvclass">)  [unwired: 7 in]
            n126 = Bundle By Name(cluster=T4 {"EventCode"=0, "Numeric"=0.0, "String"="", "Variant"=variant} ("UIMsg"), "String"=w406, "EventCode"=10) -> (w408:T4)
            n127 = call-dynamic "SaveOneSweep.vi"("Position"=w402, "SectionProperties"=w404, "error in (no error)"=w417, ".csv file from N5222A"=w406, "Temperature, deg C"=-1.0, "DataLog in"=w416) -> ("error out"=w413:errorcluster, "DataLog out"=w415:refnum<class "DataLog.lvclass">)  [unwired: 4 in]
            n128 = call-dynamic "SendUIMessage.vi"("error in (no error)"=w413, "UIMsg"=w408, "SendMessage in"=w411) -> ("error out"=w412:errorcluster, "SendMessage out"=w410:refnum<class "SendMessage.lvclass">)  [unwired: 7 in]
          }
          frame "RasterTest" {
            # "send PNA trace >>"
            n129 = call "d.vi"("error in (no error)"=w429, "ArrayController in"=w428) -> ("error out"=w430:errorcluster, "ArrayController out"=w427:refnum<class "ArrayController.lvclass">)  [unwired: 8 in]
            n130 = Unbundle By Name(w434) -> ("Position"=w431:T19[])
            n131 = flat-sequence {
              tunnel: [w451] -> w426
              tunnel: w430 -> [w451]
              frame #0 {
                n132 = Wait (ms)(milliseconds to wait=u32 10) -> ()  [unwired: 1 out]
              }
            }
            n133 = call "TriggerAndAveraging.vi"("error in (no error)"=w426, "C4209 PNA"=w444) -> ("error out"=w449:errorcluster, "C4209 PNA out"=w448:refnum<class "C4209 PNA.lvclass">)  [unwired: 8 in]
            n134 = call "SaveAndLoadTest.vi"("error in (no error)"=w449, "C4209 PNA"=w448) -> ("error out"=w447:errorcluster, "text"=w436:string, "C4209 PNA out"=w432:refnum<class "C4209 PNA.lvclass">)  [unwired: 7 in]
            n135 = Bundle By Name(cluster=T4 {"EventCode"=0, "Numeric"=0.0, "String"="", "Variant"=variant} ("UIMsg"), "String"=w436, "EventCode"=10) -> (w438:T4)
            n136 = call-dynamic "SaveOneSweep.vi"("Position"=w431, "SectionProperties"=w433, "error in (no error)"=w447, ".csv file from N5222A"=w436, "Temperature, deg C"=-1.0, "DataLog in"=w446) -> ("error out"=w443:errorcluster, "DataLog out"=w445:refnum<class "DataLog.lvclass">)  [unwired: 4 in]
            n137 = call-dynamic "SendUIMessage.vi"("error in (no error)"=w443, "UIMsg"=w438, "SendMessage in"=w441) -> ("error out"=w442:errorcluster, "SendMessage out"=w440:refnum<class "SendMessage.lvclass">)  [unwired: 7 in]
          }
          frame "Motion", "MotionFF", Default {
            # "#TBD RF off doesn't\nseem to be coded"
            # "VXM API VI inside"
            n138 = disable-structure shown="Enabled" {
              disable-tunnel: w464 -> [w478 w480]
              disable-tunnel: [w477 w480] -> w458
              disable-tunnel: [w476 _] -> w453
              frame Disabled {
                # "RF OFF"
                n139 = call "RF-Power-On-OFF.vi"("RF Power State (T: On)"=FALSE, "C4209 PNA"=w478) -> ("error out"=w476:errorcluster, "C4209 PNA out"=w477:refnum<class "C4209 PNA.lvclass">)  [unwired: 8 in]
              }
              frame Enabled {
              }
            }
            n140 = Unbundle By Name(w457) -> ("Position"=w456:T19[], "TR Module/Raster"=w455:i32, "Polarization"=w454:T17)
            n141 = call "Send Position Command.vi"("Polarization"=w454, "error in (no error)"=w453, "TR Module/Raster num"=w455, "Moves"=w456, "MotionComm in"=w460) -> ("error out"=w461:errorcluster, "MotionComm out"=w459:refnum<class "MotionComm.lvclass">)  [unwired: 5 in]
            n142 = disable-structure shown="Enabled" {
              disable-tunnel: [w472 w474] -> w466
              disable-tunnel: [w471 w475] -> w463
              disable-tunnel: w461 -> [w470 w474]
              disable-tunnel: w458 -> [w469 w475]
              frame Disabled {
                # "RF ON"
                n143 = call "RF-Power-On-OFF.vi"("error in (no error)"=w470, "RF Power State (T: On)"=TRUE, "C4209 PNA"=w469) -> ("error out"=w472:errorcluster, "C4209 PNA out"=w471:refnum<class "C4209 PNA.lvclass">)  [unwired: 7 in]
              }
              frame Enabled {
              }
            }
          }
          frame "SeqComplete" {
            n144 = call-dynamic "CloseFile.vi"("error in (no error)"=w490, "DataLog in"=w489) -> ("error out"=w487:errorcluster, "DataLog out"=w488:refnum<class "DataLog.lvclass">)  [unwired: 8 in]
            n145 = call "RF-Power-On-OFF.vi"("error in (no error)"=w487, "RF Power State (T: On)"=FALSE, "C4209 PNA"=w485) -> ("error out"=w483:errorcluster, "C4209 PNA out"=w484:refnum<class "C4209 PNA.lvclass">)  [unwired: 7 in]
          }
        }
        n146 = case shown="True" w382 {
          tunnel: [w495 w497] -> w396
          tunnel: w395 -> [w494 _]
          tunnel: w380 -> [w493 w497]
          frame False {
            n147 = call "Enque(CommandOnly).vi"("error in"=w493, "Message Command"="TestSequence" ("Command"), "Message que"=w494) -> ("error out"=w495:errorcluster)  [unwired: 7 in, 1 out]
          }
          frame True {
          }
        }
        n148 = Bundle By Name(cluster=w392, "Sequence"=w389, "AC"=w388, "PNA"=w386, "DataLog"=w379, "UI Msg"=w376, "Motion ACK"=w374) -> (w391:T3)
      }
      frame "TestSeqPause" {
        n149 = Unbundle By Name(w502) -> ("Sequence"=w501:refnum<class "Sequence.lvclass">)
        n150 = call "Pause.vi"("error in (no error)"=w500, "Sequence in"=w501) -> ("error out"=w506:errorcluster, "SeqPaused"=w498:bool, "Sequence out"=w503:refnum<class "Sequence.lvclass">)  [unwired: 7 in]
        n151 = case shown="True" w498 {
          tunnel: [w507 w509] -> w505
          tunnel: w506 -> [w507 w510]
          tunnel: w499 -> [_ w508]
          frame False {
          }
          frame True {
            # "state becomes idle"
            n152 = Flush Queue(queue=w508, error in (no error)=w510) -> (error out=w509:errorcluster)  [unwired: 2 out]
          }
        }
        n153 = Bundle By Name(cluster=w502, "Sequence"=w503) -> (w504:T3)
      }
      frame "TestSeqResume" {
        n154 = Unbundle By Name(w517) -> ("Sequence"=w516:refnum<class "Sequence.lvclass">)
        n155 = call "Resume.vi"("error in (no error)"=w515, "Sequence in"=w516) -> ("error out"=w511:errorcluster, "TestSeqResumed"=w513:bool, "Sequence out"=w518:refnum<class "Sequence.lvclass">)  [unwired: 7 in]
        n156 = case shown="True" w513 {
          tunnel: [w520 w523] -> w514
          tunnel: w512 -> [_ w522]
          tunnel: w511 -> [w520 w521]
          frame False {
          }
          frame True {
            n157 = call "Enque(CommandOnly).vi"("error in"=w521, "Message Command"="TestSequence" ("Command"), "Message que"=w522) -> ("error out"=w523:errorcluster)  [unwired: 7 in, 1 out]
          }
        }
        n158 = Bundle By Name(cluster=w517, "Sequence"=w518) -> (w519:T3)
      }
      frame "TestSeqStop" {
        # "resume\nexecution"
        n159 = Unbundle By Name(w534) -> ("Sequence"=w531:refnum<class "Sequence.lvclass">)
        n160 = call "Stop.vi"("error in (no error)"=w532, "Sequence in"=w531) -> ("error out"=w528:errorcluster, "Sequence out"=w530:refnum<class "Sequence.lvclass">)  [unwired: 8 in]
        n161 = Flush Queue(queue=w526, error in (no error)=w528) -> (queue out=w525:T2, error out=w527:errorcluster)  [unwired: 1 out]
        n162 = Bundle By Name(cluster=w534, "Sequence"=w530) -> (w535:T3)
        n163 = call "Enque(CommandOnly).vi"("error in"=w527, "Message Command"="TestSequence" ("Command"), "Message que"=w525) -> ("error out"=w533:errorcluster)  [unwired: 7 in, 1 out]
      }
      frame "Restart" {
        # "load config data, init resources, etc."
        n164 = Flush Queue(queue=w536, error in (no error)=w537) -> (queue out=w539:T2, error out=w544:errorcluster)  [unwired: 1 out]
        n165 = call "Enque(CommandOnly).vi"("error in"=w544, "Message Command"="Stop_Close" ("Command"), "Message que"=w539) -> ("error out"=w543:errorcluster, "Message que out"=w541:T2)  [unwired: 7 in]
        n166 = call "Enque(CommandOnly).vi"("error in"=w543, "Message Command"="Start" ("Command"), "Message que"=w541) -> ("error out"=w538:errorcluster)  [unwired: 7 in, 1 out]
      }
      frame "Test" {
        # "should generate error if\nsettings or hardware are wrong"
      }
      frame "AC_Reset" {
        n167 = Unbundle By Name(w551) -> ("AC"=w552:refnum<class "ArrayController.lvclass">)
        n168 = call "Reset.vi"("error in (no error)"=w547, "ArrayController in"=w552) -> ("error out"=w548:errorcluster, "ArrayController out"=w549:refnum<class "ArrayController.lvclass">)  [unwired: 8 in]
        n169 = Bundle By Name(cluster=w551, "AC"=w549) -> (w550:T3)
      }
      frame "AC_Temperature" {
        n170 = call "ConvertTo(DBL).vi"("error in"=w563, "Message Payload"=w562) -> ("error out"=w554:errorcluster, "Message Payload DBL Numeric"=w553:dbl)  [unwired: 8 in]
        n171 = Unbundle By Name(w565) -> ("UI Msg"=w557:refnum<class "SendMessage.lvclass">, "AC"=w555:refnum<class "ArrayController.lvclass">)
        n172 = Bundle By Name(cluster=T4 {"EventCode"=0, "Numeric"=0.0, "String"="", "Variant"=variant} ("UIMsg"), "EventCode"=8, "Numeric"=w553) -> (w558:T4)
        n173 = call-dynamic "SendUIMessage.vi"("error in (no error)"=w554, "UIMsg"=w558, "SendMessage in"=w557) -> ("error out"=w561:errorcluster, "SendMessage out"=w556:refnum<class "SendMessage.lvclass">)  [unwired: 7 in]
        n174 = Bundle By Name(cluster=w565, "AC"=w555, "UI Msg"=w556) -> (w564:T3)
      }
      frame "AC_d" {
        n175 = call "ConvertTo(waveform).vi"("error in"=w570, "Message Payload"=w574) -> ("error out"=w571:errorcluster, "d Cmd Payload"=w573:T16)  [unwired: 8 in]
        n176 = Unbundle By Name(w569) -> ("AC"=w572:refnum<class "ArrayController.lvclass">)
        n177 = call "d.vi"("error in (no error)"=w571, "d Cmd Properties"=w573, "ArrayController in"=w572) -> ("error out"=w566:errorcluster, "ArrayController out"=w567:refnum<class "ArrayController.lvclass">)  [unwired: 7 in]
        n178 = Bundle By Name(cluster=w569, "AC"=w567) -> (w568:T3)
      }
      frame "N5222A_Sweep" {
        n179 = Unbundle By Name(w577) -> ("PNA"=w575:refnum<class "C4209 PNA.lvclass">)
        n180 = Bundle By Name(cluster=w577, "PNA"=w575) -> (w576:T3)
      }
      frame "Stop_Close" {
        # "ignore errors"
        n181 = Unbundle By Name(w586) -> ("AC"=w583:refnum<class "ArrayController.lvclass">, "PNA"=w584:refnum<class "C4209 PNA.lvclass">)
        n182 = call "Close.vi"("C4209 PNA"=w584) -> ("error out"=w581:errorcluster, "C4209 PNA out"=w580:refnum<class "C4209 PNA.lvclass">)  [unwired: 9 in]
        n183 = call "Close.vi"("ArrayController in"=w583) -> ("error out"=w582:errorcluster, "ArrayController out"=w579:refnum<class "ArrayController.lvclass">)  [unwired: 9 in]
        n184 = flat-sequence {
          tunnel: w582 -> [_]
          tunnel: w581 -> [_]
          frame #0 {
          }
        }
        n185 = Bundle By Name(cluster=w586, "PNA"=w580, "AC"=w579) -> (w585:T3)
      }
      frame "GenerateTestError" {
        n186 = call "ConvertTo(error).vi"("Message Payload"=w587) -> ("Message Payload error"=w588:errorcluster)  [unwired: 9 in, 1 out]
      }
      frame "ExitNow" {
      }
    }
    "error out" <- w24
    n187 = call "SendErrorMessageToErrorLoop.vi"("Error Message que"=w23, "error in (no error)"=w24, "Loop Message que"=w22) -> ()  [unwired: 8 in, 1 out]
    "i" <- w26
  }
  n188 = Release Queue(queue=w13) -> ()  [unwired: 2 in, 3 out]
